vi "process_averager.vi"() -> ()   [LabVIEW 2011, in "Fiberscope_library.lvlib"]
uses:
  Fiberscope_library.lvlib
  typedefs/control_process_state_cluster.ctl
  typedefs/control_process_state_enum.ctl
  typedefs/element_images_cluster.ctl
  typedefs/feedback_to_watchdog.ctl
  typedefs/feedback_from_process_enum.ctl
panel:
  out "Averages per frame":u8
  out "Average":u8
  out "error out":errorcluster
  in  "error in":errorcluster
  # "of"
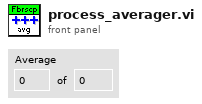
[diagram p1: front panel]
types:
  T1 = typedef "Fiberscope_library.lvlib/feedback_to_watchdog.ctl" = cluster{"Feedback_from_process_enum":T2, "Process_name":string}
  T2 = typedef "Fiberscope_library.lvlib/feedback_from_process_enum.ctl" = enum16{"Has_initialised", "Changed_parameters", "Has_started", "Has_stopped", "Has_quitted", "Is_running", "Has_finished", "Custom"}
  T3 = typedef "Fiberscope_library.lvlib/element_images_cluster.ctl" = cluster{"Images_array":dbl[][][], "#channels":i32, "Last element?":bool}
  T4 = typedef "Fiberscope_library.lvlib/control_process_state_cluster.ctl" = cluster{"Control_process_state_enum":T5, "variant":variant}
  T5 = typedef "Fiberscope_library.lvlib/control_process_state_enum.ctl" = enum16{"Init", "Quit", "Start", "Stop", "Change_parameters", "Running", "Finish", "Custom"}
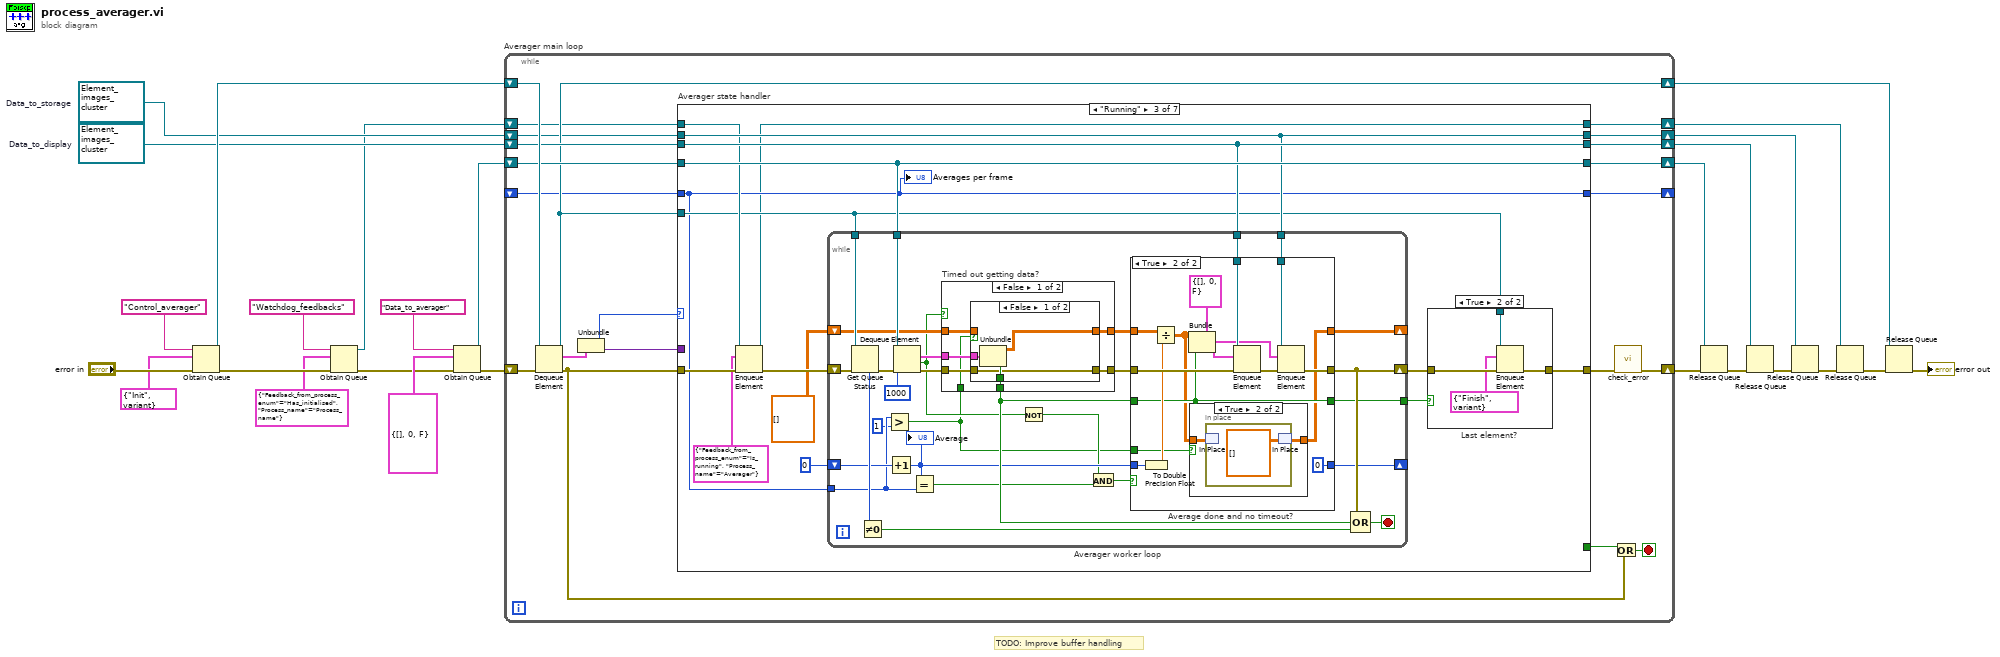
[diagram p0: block diagram]
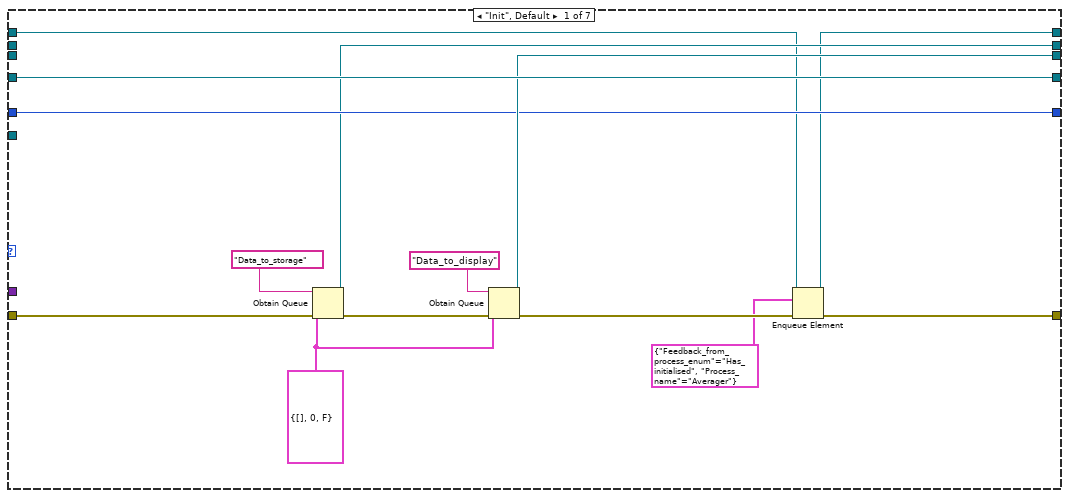
[diagram p2: hidden frame]
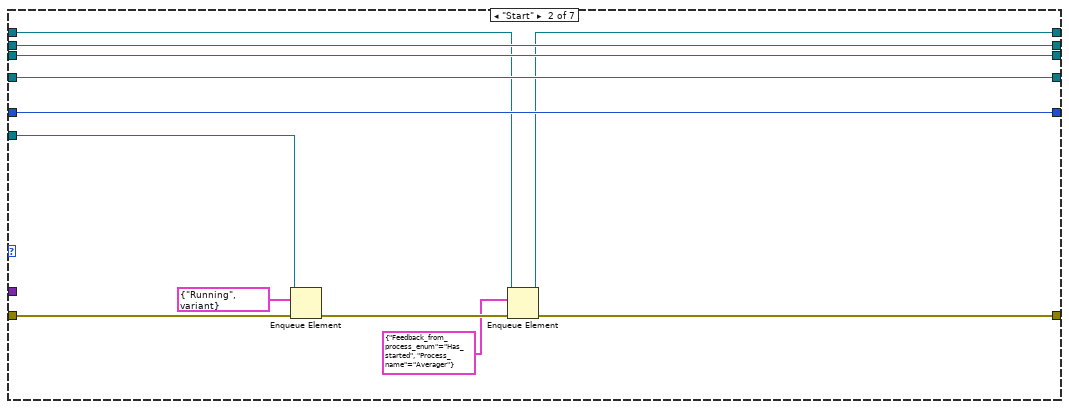
[diagram p3: hidden frame]
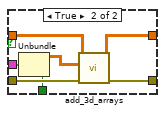
[diagram p7: hidden frame]
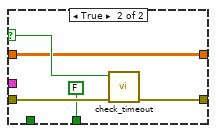
[diagram p8: hidden frame]
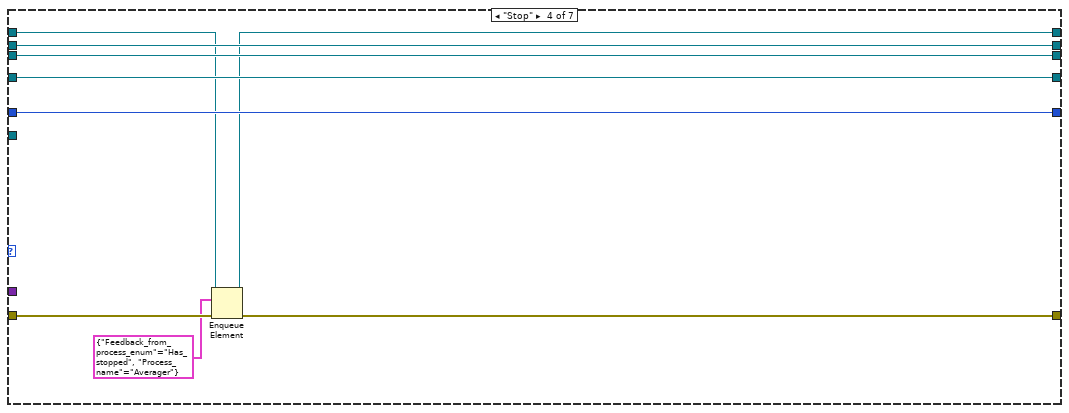
[diagram p9: hidden frame]
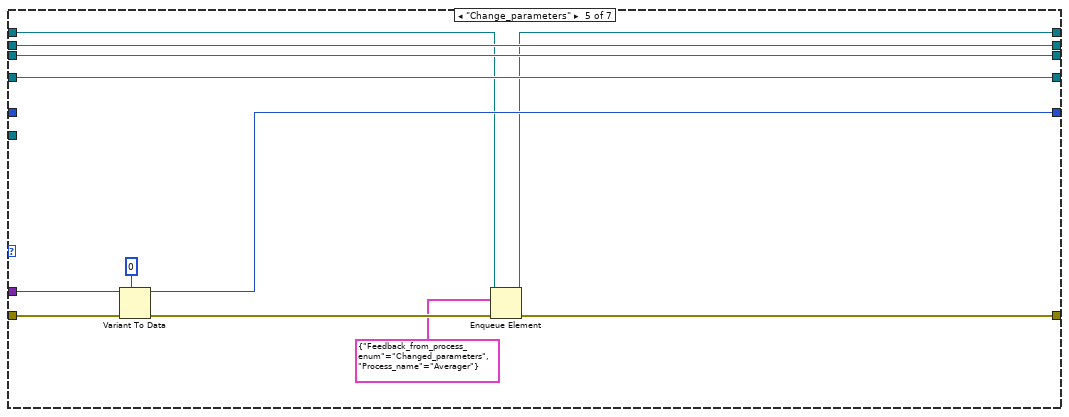
[diagram p10: hidden frame]
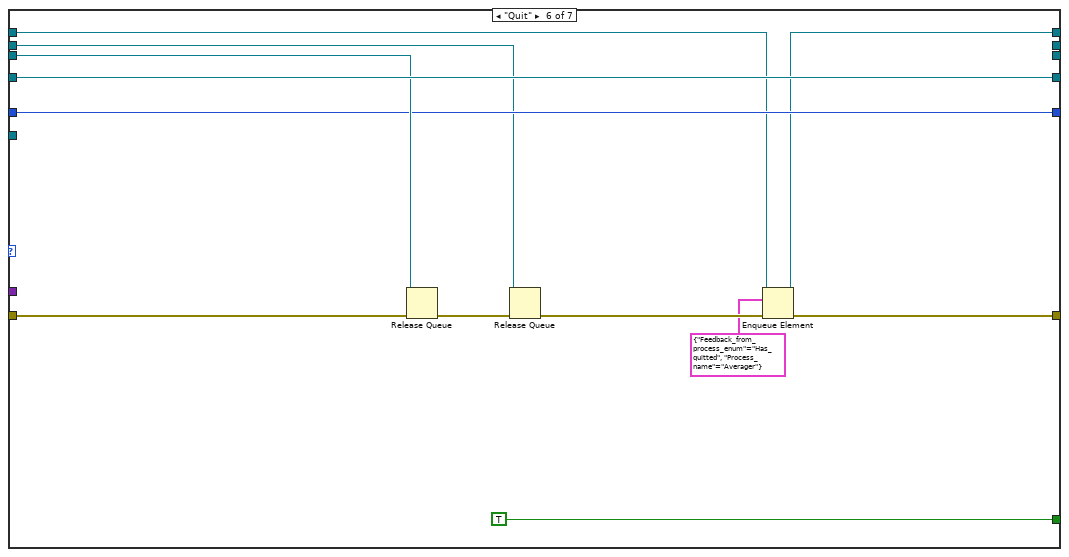
[diagram p11: hidden frame]
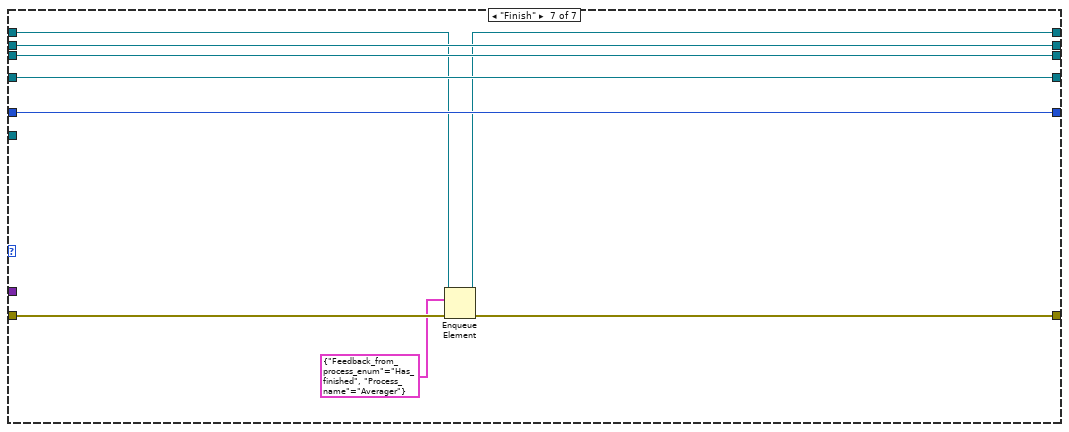
[diagram p12: hidden frame]
diagram:
  w6 = refnum<queue> refnum  # Data_to_display
  w7 = refnum<queue> refnum  # Data_to_storage
  # "TODO: Improve buffer handling"
  n1 = Obtain Queue(name (unnamed)="Control_averager", element data type=T4 {"Control_process_state_enum"=enum."Init", "variant"=variant} ("Control_process_state_cluster"), error in (no error)="error in") -> (queue out=w21:refnum<queue>, error out=w5:errorcluster)  [unwired: 2 in, 1 out]
  n2 = Obtain Queue(name (unnamed)="Watchdog_feedbacks", element data type=T1 {"Feedback_from_process_enum"=enum."Has_initialised", "Process_name"="Process_name"}, error in (no error)=w5) -> (queue out=w2:refnum<queue>, error out=w4:errorcluster)  [unwired: 2 in, 1 out]
  n3 = Obtain Queue(name (unnamed)="Data_to_averager", element data type=T3 {"Images_array"=[], "#channels"=0, "Last element?"=FALSE} ("Element_images_cluster"), error in (no error)=w4) -> (queue out=w20:refnum<queue>, error out=w22:errorcluster)  [unwired: 2 in, 1 out]
  n4 = while "Averager main loop" {
    shift-right: [w38] -> w19
    shift-left: w22 -> [w47]
    shift-right: [w35] -> w17
    shift-left: w21 -> [w46]
    shift-right: [w42] -> w18
    shift-left: w20 -> [w43]
    shift-right: [w40] -> w13
    shift-left: w6 -> [w41]
    shift-right: [w34] -> _
    shift-left: _ -> [w33]
    shift-right: [w31] -> w12
    shift-left: w7 -> [w32]
    shift-right: [w27] -> w8
    shift-left: w2 -> [w28]
    stop <- w37 stop-if-true
    n5 = Dequeue Element(queue=w46, error in (no error)=w47) -> (queue out=w35:refnum<queue>, element=w45:T4, error out=w29:errorcluster)  [unwired: 1 in, 1 out]
    n6 = Unbundle(w45) -> ("Control_process_state_enum"=w44:T5, "variant"=w36:variant)
    n7 = case "Averager state handler" shown="\"Running\"" w44 {
      tunnel: w29 -> [w56 w68 w85 w172 w186 w197 w205]
      tunnel: [w52 w67 w81 w171 w180 w192 w204] -> w39
      tunnel: w43 -> [w61 w73 w88 w176 w188 w200 w209]
      tunnel: [w61 w73 w88 w176 w188 w200 w209] -> w42
      tunnel: w41 -> [_ w72 w87 w175 w187 w198 w208]
      tunnel: [w59 w72 w87 w175 w187 _ w208] -> w40
      tunnel: [_ _ _ _ _ TRUE _] -> w30
      tunnel: w36 -> [_ _ _ _ w185 _ _]
      tunnel: w35 -> [_ w66 w80 _ _ _ _]
      tunnel: [w58 w71 w77 w174 w184 w196 w207] -> w34
      tunnel: w33 -> [w58 w71 w77 w174 _ w196 w207]
      tunnel: w32 -> [_ w70 w86 w173 w183 w194 w206]
      tunnel: [w54 w70 w86 w173 w183 _ w206] -> w31
      tunnel: w28 -> [w51 w64 w83 w170 w179 w191 w203]
      tunnel: [w49 w63 w75 w169 w178 w190 w202] -> w27
      frame "Init", Default {
        w50 = T3 {"Images_array"=[], "#channels"=0, "Last element?"=FALSE} ("Element_images_cluster")
        n8 = Obtain Queue(name (unnamed)="Data_to_storage", element data type=w50, error in (no error)=w56) -> (queue out=w54:refnum<queue>, error out=w55:errorcluster)  [unwired: 2 in, 1 out]
        n9 = Obtain Queue(name (unnamed)="Data_to_display", element data type=w50, error in (no error)=w55) -> (queue out=w59:refnum<queue>, error out=w53:errorcluster)  [unwired: 2 in, 1 out]
        n10 = Enqueue Element(queue=w51, element=T1 {"Feedback_from_process_enum"=enum."Has_initialised", "Process_name"="Averager"}, error in (no error)=w53) -> (queue out=w49:refnum<queue>, error out=w52:errorcluster)  [unwired: 1 in, 1 out]
      }
      frame "Start" {
        n11 = Enqueue Element(queue=w66, element=T4 {"Control_process_state_enum"=enum."Running", "variant"=variant}, error in (no error)=w68) -> (error out=w69:errorcluster)  [unwired: 1 in, 2 out]
        n12 = Enqueue Element(queue=w64, element=T1 {"Feedback_from_process_enum"=enum."Has_started", "Process_name"="Averager"}, error in (no error)=w69) -> (queue out=w63:refnum<queue>, error out=w67:errorcluster)  [unwired: 1 in, 1 out]
      }
      frame "Running" {
        n13 = Enqueue Element(queue=w83, element=T1 {"Feedback_from_process_enum"=enum."Is_running", "Process_name"="Averager"}, error in (no error)=w85) -> (queue out=w75:refnum<queue>, error out=w84:errorcluster)  [unwired: 1 in, 1 out]
        n14 = while "Averager worker loop" {
          shift-right: [w104] -> w82
          shift-left: w84 -> [w122]
          tunnel: w80 -> [w121]
          tunnel: w88 -> [w120]
          tunnel: w87 -> [w117]
          tunnel: w86 -> [w115]
          shift-right: [w102] -> _
          shift-left: dbl[][][] [] -> [w106]
          tunnel: w77 -> [w96]
          shift-right: [w103] -> _
          shift-left: u8 0 -> [w107]
          tunnel: [w97] -> w76
          stop <- w116 stop-if-true
          n15 = Get Queue Status(queue=w121, error in (no error)=w122) -> (error out=w113:errorcluster, # elements in queue=w109:i32)  [unwired: 1 in, 6 out]
          n16 = Not Equal To 0?(x=w109) -> (x != 0?=w108:bool)
          n17 = Greater?(x=w96, y=u8 1) -> (0:w94:bool)
          n18 = Increment(x=w107) -> (x+1=w105:u8)
          "Average" <- w105
          n19 = Dequeue Element(queue=w120, timeout in ms (-1)=1000, error in (no error)=w113) -> (element=w110:T3, timed out?=w99:bool, error out=w111:errorcluster)  [unwired: 1 out]
          n20 = Equal?(x=w105, y=w96) -> (x = y?=w101:bool)
          n21 = case "Timed out getting data?" shown="False" w99 {
            selector: w99 -> [_ w165]
            tunnel: w111 -> [w151 w167]
            tunnel: [w150 w166] -> w119
            tunnel: w110 -> [w147 _]
            tunnel: [w148 w164] -> w118
            tunnel: w106 -> [w149 w164]
            tunnel: [w146 FALSE ("Last element?")] -> w114
            tunnel: w94 -> [w145 _]
            frame False {
              n22 = case shown="False" w145 {
                tunnel: w151 -> [w152 w162]
                tunnel: [w152 w161] -> w150
                tunnel: w149 -> [_ w160]
                tunnel: [w153 w159] -> w148
                tunnel: w147 -> [w155 w158]
                tunnel: [w154 w156] -> w146
                frame False {
                  n23 = Unbundle(w155) -> ("Images_array"=w153:dbl[][][], "Last element?"=w154:bool)  [unwired: 1 out]
                }
                frame True {
                  n24 = Unbundle(w158) -> ("Images_array"=w157:dbl[][][], "Last element?"=w156:bool)  [unwired: 1 out]
                  n25 = call "add_3d_arrays.vi"("error in"=w162, "3d array in 2"=w157, "3d arry in 1"=w160) -> ("error out"=w161:errorcluster, "3d array sum out"=w159:dbl[][][])  [unwired: 5 in]
                }
              }
            }
            frame True {
              n26 = call "check_timeout.vi"("error in"=w167, "Timeout?"=w165) -> ("error out"=w166:errorcluster)  [unwired: 9 in]
            }
          }
          n27 = Not(x=w99) -> (.not. x?=w98:bool)
          n28 = And(x=w98, y=w101) -> (x .and. y?=w100:bool)
          n29 = case "Average done and no timeout?" shown="True" w100 {
            tunnel: w119 -> [w126 w141]
            tunnel: w118 -> [w125 w140]
            tunnel: w117 -> [_ w139]
            tunnel: [w126 w136] -> w104
            tunnel: w115 -> [_ w135]
            tunnel: w114 -> [w123 w130]
            tunnel: w105 -> [w124 w132]
            tunnel: [w124 u8 0 ("t")] -> w103
            tunnel: [w125 w128] -> w102
            tunnel: [w123 w130] -> w97
            tunnel: w94 -> [_ w127]
            frame False {
            }
            frame True {
              n30 = To Double Precision Float(number=w132) -> (double precision float=w138:dbl)
              n31 = Divide(x=w140, y=w138) -> (x/y=w129:dbl[][][])
              n32 = Bundle(cluster=T3 {"Images_array"=[], "#channels"=0, "Last element?"=FALSE} ("Element_images_cluster"), "Images_array"=w129, "Last element?"=w130) -> (w133:T3)  [unwired: 1 in]
              n33 = case shown="True" w127 {
                tunnel: w129 -> [_ w143]
                tunnel: [_ w142] -> w128
                frame False {
                }
                frame True {
                  n34 = in-place {
                    n35 = in-place-match #1(w143) -> ()  [unwired: 1 out]
                    n36 = in-place-match #1(dbl[][][] []) -> (w142:dbl[][][])
                  }
                }
              }
              n37 = Enqueue Element(queue=w139, element=w133, error in (no error)=w141) -> (error out=w137:errorcluster)  [unwired: 1 in, 2 out]
              n38 = Enqueue Element(queue=w135, element=w133, error in (no error)=w137) -> (error out=w136:errorcluster)  [unwired: 1 in, 2 out]
            }
          }
          n39 = Compound Arithmetic op=OR(w104, w114, w108) -> (w116:bool)
        }
        n40 = case "Last element?" shown="True" w76 {
          tunnel: w82 -> [w89 w92]
          tunnel: [w89 w93] -> w81
          tunnel: w80 -> [_ w91]
          frame False {
          }
          frame True {
            n41 = Enqueue Element(queue=w91, element=T4 {"Control_process_state_enum"=enum."Finish", "variant"=variant} ("Control_process_state_cluster"), error in (no error)=w92) -> (error out=w93:errorcluster)  [unwired: 1 in, 2 out]
          }
        }
        "Averages per frame" <- w77
      }
      frame "Stop" {
        n42 = Enqueue Element(queue=w170, element=T1 {"Feedback_from_process_enum"=enum."Has_stopped", "Process_name"="Averager"}, error in (no error)=w172) -> (queue out=w169:refnum<queue>, error out=w171:errorcluster)  [unwired: 1 in, 1 out]
      }
      frame "Change_parameters" {
        n43 = Variant To Data(error in=w186, type=u8 0 ("Averages per frame"), Variant=w185) -> (data=w184:u8, error out=w181:errorcluster)
        n44 = Enqueue Element(queue=w179, element=T1 {"Feedback_from_process_enum"=enum."Changed_parameters", "Process_name"="Averager"}, error in (no error)=w181) -> (queue out=w178:refnum<queue>, error out=w180:errorcluster)  [unwired: 1 in, 1 out]
      }
      frame "Quit" {
        n45 = Release Queue(queue=w198, error in (no error)=w197) -> (error out=w195:errorcluster)  [unwired: 1 in, 2 out]
        n46 = Release Queue(queue=w194, error in (no error)=w195) -> (error out=w193:errorcluster)  [unwired: 1 in, 2 out]
        n47 = Enqueue Element(queue=w191, element=T1 {"Feedback_from_process_enum"=enum."Has_quitted", "Process_name"="Averager"}, error in (no error)=w193) -> (queue out=w190:refnum<queue>, error out=w192:errorcluster)  [unwired: 1 in, 1 out]
      }
      frame "Finish" {
        n48 = Enqueue Element(queue=w203, element=T1 {"Feedback_from_process_enum"=enum."Has_finished", "Process_name"="Averager"}, error in (no error)=w205) -> (queue out=w202:refnum<queue>, error out=w204:errorcluster)  [unwired: 1 in, 1 out]
      }
    }
    n49 = Or(x=w30, y=w29) -> (x .or. y?=w37:bool)
    n50 = call "check_error.vi"("error in"=w39) -> ("error out"=w38:errorcluster)  [unwired: 10 in]
  }
  n51 = Release Queue(queue=w18, error in (no error)=w19) -> (error out=w15:errorcluster)  [unwired: 1 in, 2 out]
  n52 = Release Queue(queue=w13, error in (no error)=w15) -> (error out=w14:errorcluster)  [unwired: 1 in, 2 out]
  n53 = Release Queue(queue=w12, error in (no error)=w14) -> (error out=w10:errorcluster)  [unwired: 1 in, 2 out]
  n54 = Release Queue(queue=w8, error in (no error)=w10) -> (error out=w9:errorcluster)  [unwired: 1 in, 2 out]
  n55 = Release Queue(queue=w17, error in (no error)=w9) -> (error out=→"error out":errorcluster)  [unwired: 1 in, 2 out]
